vi "aparExecution_ModularLoop.vi"(9 "Motion Cfg File path":path=path "C:/Users/Public/Documents/UCAR/APAR Board Test/SupportFiles/Motion64.ini", 10 "Cfg File path":path=path "C:/Users/Public/Documents/UCAR/APAR Board Test/SupportFiles/aparConfig.ini", 11 "MessageQues":T1) -> ()   [LabVIEW 2017]
doc: "This VI is a simple state machine that has a message que so it can be controlled by external processes.\nIt also has a control with all the messages ques in the calling application that it needs to send messages to.\n\nThe concept is to have many parallel VIs like this one. This VI should be a cohesive process. This could cut down on it's size and complexity.\n\nBolder Software LLC"
uses:
  Support/MessageQue/VXM Main Test App/MultipleMessageQues vxm.ctl
  Support/MessageQue/MessageQue.ctl
  Support/MessageQue/MessageCluster.ctl
  Classes/aparCfg/aparCfg.lvclass
  Classes/ArrayController/ArrayController.lvclass
  Classes/N5222A PNA/N5222A PNA.lvclass
  Classes/Sequence/Sequence.lvclass
  Classes/Datalog/DataLog.lvclass
  Classes/SendMessage/SendMessage.lvclass
  Classes/MotionComm/MotionComm.lvclass
  Classes/FileMerge/FileMerge.lvclass
  C:/Users/Public/Documents/OU PAARD/mmWave_RF_Scanner/LVSource/Classes/Datalog/DataLog.lvclass
  Classes/DataLogRaster/DataLogRaster.lvclass
  Support/MessageAPI/UIMessage.ctl
  Support/MessageQue/MessageQue.lvlib
  Classes/VXMCfg/VXMCfg.lvclass
panel:
  out "Seq Step":string
  out "i":i32
  out "Command":string
  out "error out":errorcluster
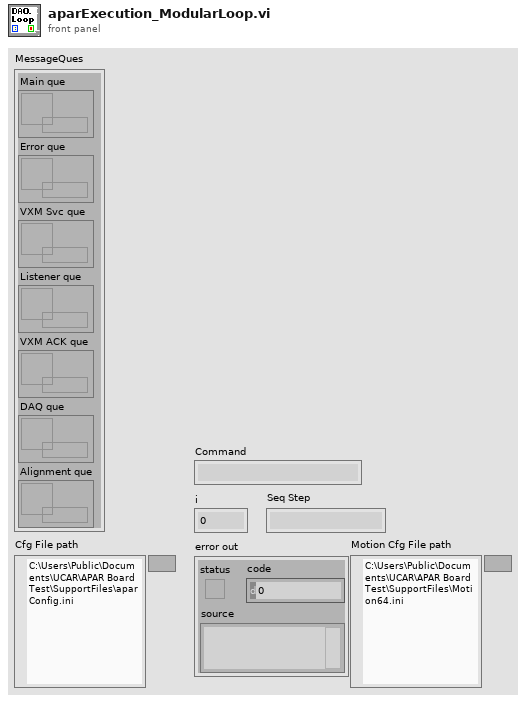
[diagram p1: front panel]
types:
  T1 = typedef "MultipleMessageQues vxm.ctl" = cluster{"Main que":T2, "Error que":T2, "VXM Svc que":T2, "Listener que":T2, "VXM ACK que":T2, "DAQ que":T2, "Alignment que":T2}
  T2 = typedef "MessageQue.lvlib/MessageQue.ctl" = refnum<queue>
  T3 = cluster{"aparCfg":refnum<class "aparCfg.lvclass">, "AC":refnum<class "ArrayController.lvclass">, "PNA":refnum<class "N5222A PNA.lvclass">, "Sequence":refnum<class "Sequence.lvclass">, "DataLog":refnum<class "DataLog.lvclass">, "UI Msg":refnum<class "SendMessage.lvclass">, "Motion ACK":refnum<class "MotionComm.lvclass">}
  T4 = typedef "UIMessage.ctl" = cluster{"EventCode":i32, "Numeric":dbl, "String":string, "Variant":variant}
  T5 = typedef "ACConfig.ctl" = cluster{"ACIPAddress":string, "timeout ms":i32, "AC (Dest.) port":u16, "Enable":bool}
  T6 = typedef "N5222AConfig.ctl" = cluster{"ResourceName":string, "Enable":bool, "Channel":i32, "CalFileName":string, "MeasName":string, "TempDatFile":string, "Power, dBm":dbl, "NumPoints":i32, "Start Freq, Hz":dbl, "Stop Freq, Hz":dbl, "NumAverages":i32, "Sweep Type":i32}
  T7 = typedef "seqConfig.ctl" = cluster{"TempXMLFilePath":path, "Motion":bool}
  T8 = typedef "RunTest.ctl" = cluster{"FileNameRoot":string, "MergeFilePath":path, "Merge":bool}
  T9 = typedef "DataLogConfig.ctl" = cluster{"FilePath":path}
  T10 = cluster{"X step":dbl, "Y step":dbl, "Z step":dbl, "T step":dbl}[]
  T11 = typedef "rasterConfig.ctl" = cluster{"Nyquist, mm":dbl, "Window, cm":dbl, "Polarization, V0 H1":T12, "RF Direction Tx0":T13}
  T12 = typedef "PolarizationSelect.ctl" = enum16{"Vertical", "Horizontal"}
  T13 = typedef "RF Direction.ctl" = enum16{"Tx - RF In", "Rx - RF Out"}
  T14 = typedef "DataLog.lvclass/SearchableTag.ctl" = cluster{"Module, 0-63":i32, "RF Direction Tx0":T13, "Polarization, V0 H1":T12, "PhaseShift, deg":dbl, "Atten, dB":dbl}
  T15 = typedef "PatchNewTestStep.ctl" = cluster{"RF In/Out":T13, "TR Module/Raster":i32, "Polarization":T12, "Position":cluster{"X mm":dbl, "Y mm":dbl, "Z mm":dbl, "T deg":dbl}}
  T16 = cluster{"X mm":dbl, "Y mm":dbl, "Z mm":dbl, "T deg":dbl}
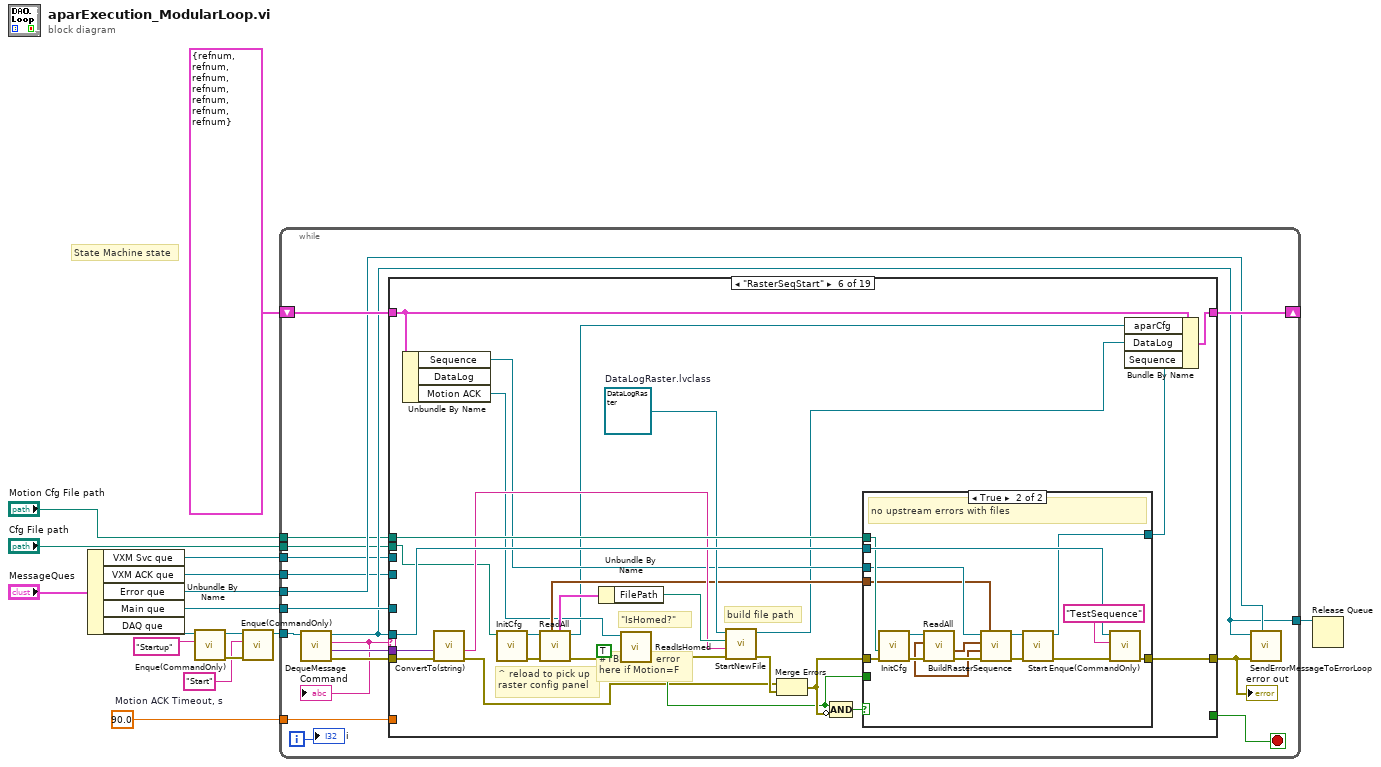
[diagram p0: block diagram]
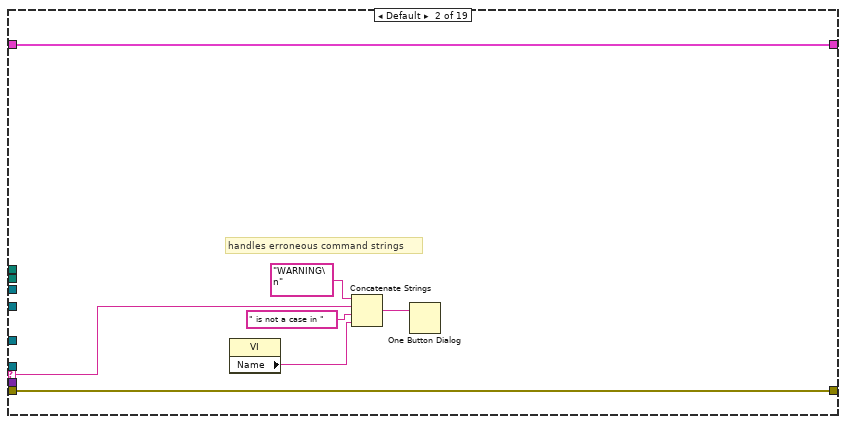
[diagram p3: hidden frame]
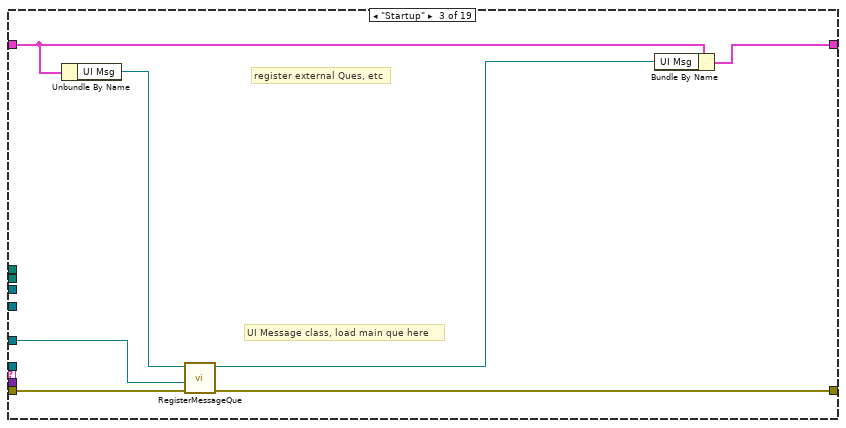
[diagram p4: hidden frame]
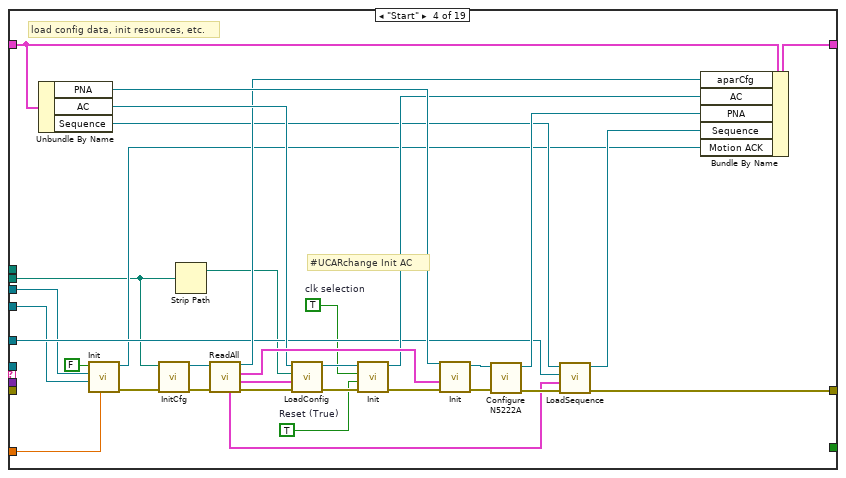
[diagram p5: hidden frame]
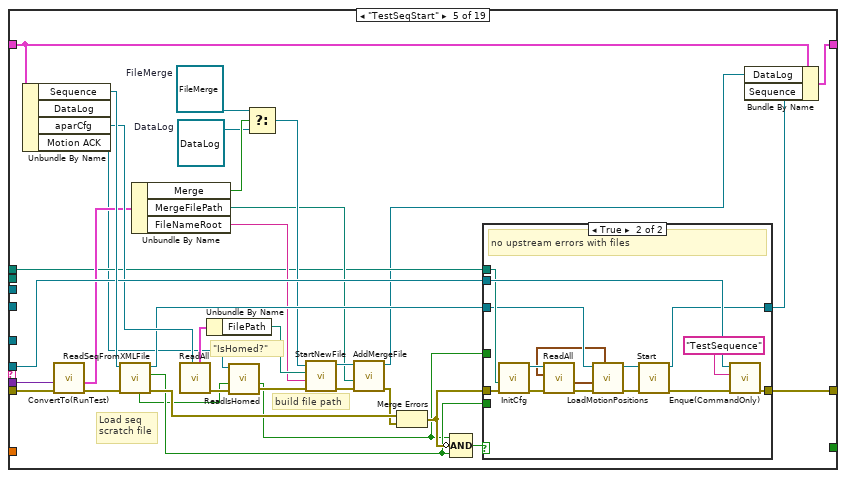
[diagram p6: hidden frame]
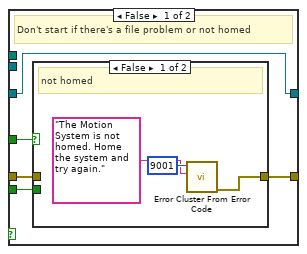
[diagram p7: hidden frame]
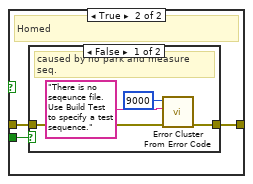
[diagram p8: hidden frame]
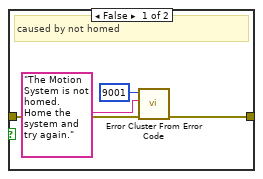
[diagram p11: hidden frame]
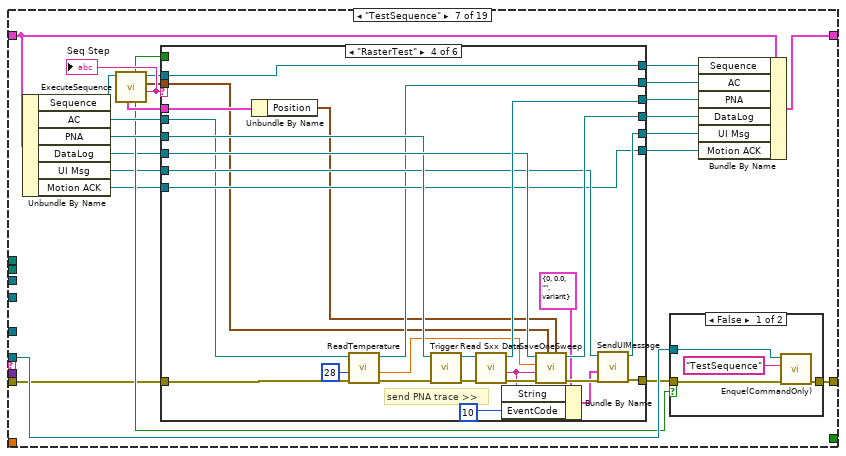
[diagram p12: hidden frame]
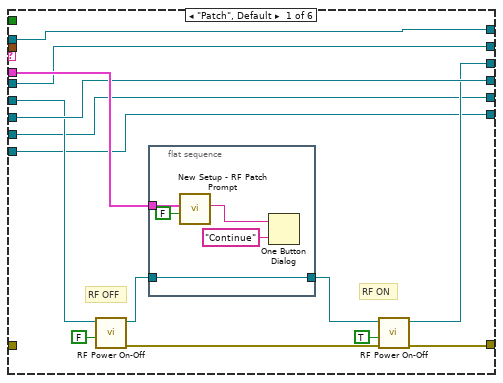
[diagram p13: hidden frame]
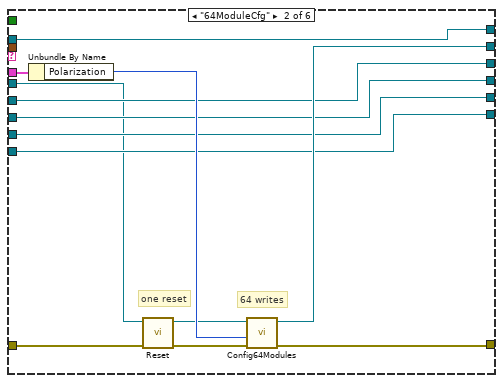
[diagram p14: hidden frame]
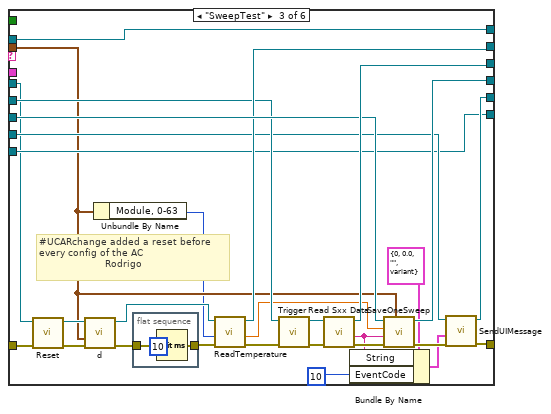
[diagram p15: hidden frame]
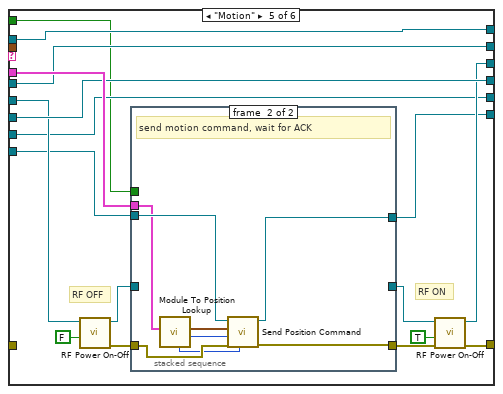
[diagram p16: hidden frame]
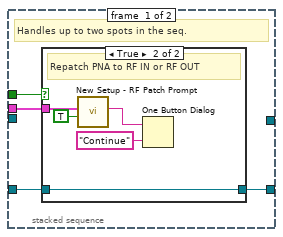
[diagram p17: hidden frame]
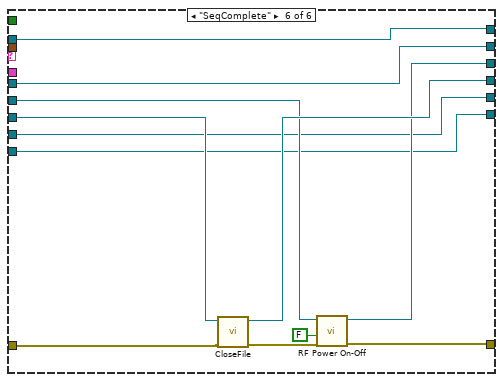
[diagram p19: hidden frame]
diagram:
  w2 = 90.0  # Motion ACK Timeout, s
  # "State Machine state"
  n1 = Unbundle By Name("MessageQues") -> ("VXM Svc que"=w4:T2, "VXM ACK que"=w3:T2, "Error que"=w14:T2, "Main que"=w15:T2, "DAQ que"=w12:T2)
  n2 = call "Enque(CommandOnly).vi"("Message Command"="Startup" ("Command"), "Message que"=w12) -> ("error out"=w9:errorcluster, "Message que out"=w8:T2)  [unwired: 8 in]
  n3 = call "Enque(CommandOnly).vi"("error in"=w9, "Message Command"="Start", "Message que"=w8) -> ("Message que out"=w7:T2)  [unwired: 7 in, 1 out]
  n4 = while {
    tunnel: w7 -> [w33]
    tunnel: w15 -> [w32]
    tunnel: w14 -> [w23]
    tunnel: [w22] -> w13
    shift-right: [w28] -> _
    shift-left: T3 {"aparCfg"=refnum, "AC"=refnum, "PNA"=refnum, "Sequence"=refnum, "DataLog"=refnum, "UI Msg"=refnum, "Motion ACK"=refnum} -> [w27]
    tunnel: "Cfg File path" -> [w21]
    tunnel: w4 -> [w20]
    tunnel: w3 -> [w19]
    tunnel: w2 -> [w18]
    tunnel: "Motion Cfg File path" -> [w17]
    i -> [w26]
    stop <- w30 stop-if-true
    n5 = call "DequeMessage.vi"("Message que"=w33) -> ("error out"=w31:errorcluster, "Message Payload"=w29:variant, "Message Command"=w25:string, "Message que out"=w22:T2)  [unwired: 5 in, 2 out]
    "Command" <- w25
    n6 = case shown="\"RasterSeqStart\"" w25 {
      selector: w25 -> [_ w36 _ _ _ _ _ _ _ _ _ _ _ _ _ _ _ _ _]
      tunnel: w32 -> [_ _ w43 w58 _ _ _ _ _ _ _ _ _ _ _ _ _ _ _]
      tunnel: w22 -> [_ _ _ _ w113 w173 w222 w365 w379 w393 w403 _ _ _ _ _ _ _ _]
      tunnel: [_ w41 w47 w62 w115 w174 w223 w372 w381 w400 w405 _ w415 w426 w436 w448 _ w458 _] -> w24
      tunnel: w31 -> [_ w41 w42 _ w109 w169 w208 w366 w382 w399 w404 _ w414 w431 w440 w448 _ _ _]
      tunnel: [_ _ _ _ _ _ _ _ _ _ _ _ _ _ _ _ _ _ TRUE] -> w30
      tunnel: w29 -> [_ _ _ _ w110 w170 _ _ _ _ _ _ _ w430 w444 _ _ w457 _]
      tunnel: [w34 w40 w45 w72 w111 w171 w218 w370 w386 w402 w412 w413 w417 w433 w438 w446 w455 w459 w460] -> w28
      tunnel: w27 -> [w34 w40 w46 w73 w112 w172 w219 w368 w384 w401 w412 w413 w418 w434 w439 w447 w456 w459 w460]
      tunnel: w21 -> [_ _ _ w50 _ w151 _ _ _ _ _ _ _ _ _ _ _ _ _]
      tunnel: w20 -> [_ _ _ w54 _ _ _ _ _ _ _ _ _ _ _ _ _ _ _]
      tunnel: w19 -> [_ _ _ w53 _ _ _ _ _ _ _ _ _ _ _ _ _ _ _]
      tunnel: w18 -> [_ _ _ w52 _ _ _ _ _ _ _ _ _ _ _ _ _ _ _]
      tunnel: w17 -> [_ _ _ _ w88 w163 _ _ _ _ _ _ _ _ _ _ _ _ _]
      frame "idle" {
      }
      frame Default {
        # "handles erroneous command strings"
        n7 = property class="VI"() -> ("Name"=w35:string)  [unwired: 2 in, 2 out]
        n8 = Concatenate Strings("WARNING\n" ("message"), w36, " is not a case in " ("message"), w35) -> (w39:string)
        n9 = One Button Dialog(message=w39) -> ()  [unwired: 1 in, 1 out]
      }
      frame "Startup" {
        # "UI Message class, load main que here"
        # "register external Ques, etc"
        n10 = Unbundle By Name(w46) -> ("UI Msg"=w48:refnum<class "SendMessage.lvclass">)
        n11 = call "RegisterMessageQue.vi"("error in (no error)"=w42, "Message que"=w43, "SendMessage in"=w48) -> ("error out"=w47:errorcluster, "SendMessage out"=w44:refnum<class "SendMessage.lvclass">)  [unwired: 7 in]
        n12 = Bundle By Name(cluster=w46, "UI Msg"=w44) -> (w45:T3)
      }
      frame "Start" {
        w51 = TRUE  # clk selection
        w64 = TRUE  # Reset (True)
        # "#UCARchange Init AC"
        # "load config data, init resources, etc."
        n13 = Unbundle By Name(w73) -> ("PNA"=w74:refnum<class "N5222A PNA.lvclass">, "AC"=w75:refnum<class "ArrayController.lvclass">, "Sequence"=w61:refnum<class "Sequence.lvclass">)
        n14 = call "Init.vi"("Timeout, s"=w52, "VXM ACK que"=w53, "VXM Svc que"=w54, "Standalone"=FALSE) -> ("error out"=w57:errorcluster, "MotionComm out"=w56:refnum<class "MotionComm.lvclass">)  [unwired: 6 in]
        n15 = call "InitCfg.vi"("error in (no error)"=w57, "Cfg File path"=w50) -> ("error out"=w68:errorcluster, "aparCfg out"=w69:refnum<class "aparCfg.lvclass">)  [unwired: 8 in]
        n16 = Strip Path(path=w50) -> (stripped path=w49:path)  [unwired: 1 out]
        n17 = call "ReadAll.vi"("error in (no error)"=w68, "aparCfg in"=w69) -> ("error out"=w77:errorcluster, "ACConfig"=w81:T5, "N5222A Cfg"=w79:T6, "aparCfg out"=w71:refnum<class "aparCfg.lvclass">, "SequenceConfig"=w59:T7)  [unwired: 3 in, 2 out]
        n18 = call "LoadConfig.vi"("error in (no error)"=w77, "AC Config"=w81, "Support Files Path"=w49, "ArrayController in"=w75) -> ("error out"=w80:errorcluster, "ArrayController out"=w76:refnum<class "ArrayController.lvclass">)  [unwired: 6 in]
        n19 = call "Init.vi"("error in (no error)"=w80, "Reset (True)"=w64, "clk selection"=w51, "ArrayController in"=w76) -> ("error out"=w78:errorcluster, "ArrayController out"=w70:refnum<class "ArrayController.lvclass">)  [unwired: 5 in, 1 out]
        n20 = call "Init.vi"("error in (no error)"=w78, "N5222A Cfg"=w79, "N5222A PNA in"=w74) -> ("error out"=w65:errorcluster, "N5222A PNA out"=w67:refnum<class "N5222A PNA.lvclass">)  [unwired: 7 in]
        n21 = call "Configure N5222A.vi"("error in (no error)"=w65, "N5222A PNA in"=w67) -> ("error out"=w63:errorcluster, "N5222A PNA out"=w66:refnum<class "N5222A PNA.lvclass">)  [unwired: 8 in]
        n22 = call "LoadSequence.vi"("error in (no error)"=w63, "Sequence Cfg"=w59, "Message que"=w58, "Sequence in"=w61) -> ("error out"=w62:errorcluster, "Sequence out"=w60:refnum<class "Sequence.lvclass">)  [unwired: 6 in]
        n23 = Bundle By Name(cluster=w73, "aparCfg"=w71, "AC"=w70, "PNA"=w66, "Sequence"=w60, "Motion ACK"=w56) -> (w72:T3)
      }
      frame "TestSeqStart" {
        w96 = refnum<class "FileMerge.lvclass"> refnum  # FileMerge
        w95 = refnum<class "DataLog.lvclass"> refnum  # DataLog
        # "\"IsHomed?\""
        # "build file path"
        # "Load seq \nscratch file"
        n24 = Unbundle By Name(w112) -> ("Sequence"=w114:refnum<class "Sequence.lvclass">, "aparCfg"=w107:refnum<class "aparCfg.lvclass">, "Motion ACK"=w84:refnum<class "MotionComm.lvclass">)  [unwired: 1 out]
        n25 = call "ConvertTo(RunTest).vi"("error in"=w109, "Message Payload"=w110) -> ("error out"=w108:errorcluster, "RunTest"=w106:T8)  [unwired: 8 in]
        n26 = call "ReadSeqFromXMLFile.vi"("error in (no error)"=w108, "Sequence in"=w114) -> ("error out"=w103:errorcluster, "Valid Seq"=w99:bool, "Sequence out"=w102:refnum<class "Sequence.lvclass">, "Motion"=w82:bool)  [unwired: 5 in, 1 out]
        n27 = Unbundle By Name(w106) -> ("Merge"=w97:bool, "MergeFilePath"=w89:path, "FileNameRoot"=w90:string)
        n28 = call "ReadAll.vi"("aparCfg in"=w107) -> ("error out"=w86:errorcluster, "DataLogConfig"=w105:T9)  [unwired: 4 in, 5 out]
        n29 = Unbundle By Name(w105) -> ("FilePath"=w104:path)
        n30 = call "ReadIsHomed.vi"("error in (no error)"=w86, "Motion Config"=w82, "MotionComm in"=w84) -> ("error out"=w85:errorcluster, "True = Homed"=w83:bool)  [unwired: 6 in, 1 out]
        n31 = Select(t=w96, s=w97, f=w95) -> (s? t:f=w94:refnum<class "DataLog.lvclass">)
        n32 = call-dynamic "StartNewFile.vi"("error in (no error)"=w85, "Root File Name"=w90, "Data Files Folder Path"=w104, "DataLog in"=w94) -> ("error out"=w93:errorcluster, "DataLog out"=w91:refnum<class "DataLog.lvclass">)  [unwired: 6 in]
        n33 = call-dynamic "AddMergeFile.vi"("error in (no error)"=w93, "ExistingFilePath"=w89, "DataLog in"=w91) -> ("error out"=w92:errorcluster, "DataLog out"=w87:refnum<class "DataLog.lvclass">)  [unwired: 7 in]
        n34 = Merge Errors(w103, w92) -> (w101:errorcluster)
        n35 = Compound Arithmetic op=AND(w83, invert w101, w99) -> (w100:bool)
        n36 = case shown="True" w100 {
          tunnel: [w119 w146] -> w115
          tunnel: w113 -> [_ w145]
          tunnel: w101 -> [w120 w140]
          tunnel: w102 -> [w117 w134]
          tunnel: [w117 w142] -> w98
          tunnel: w99 -> [w118 _]
          tunnel: w88 -> [_ w138]
          tunnel: w83 -> [w116 _]
          frame False {
            # "Don't start if there's a file problem or not homed"
            n37 = case shown="False" w116 {
              tunnel: w120 -> [_ w126]
              tunnel: [w121 w125] -> w119
              tunnel: w118 -> [_ w124]
              frame False {
                # "not homed"
                n38 = call <vilib>:"Error Cluster From Error Code.vi"("error message (\"\")"="The Motion System is not homed. Home the system and try again." ("error message (\"\")"), "error code (0)"=9001) -> ("error out"=w121:errorcluster)  [unwired: 7 in]
              }
              frame True {
                # "Homed"
                n39 = case shown="False" w124 {
                  tunnel: w126 -> [w130 w131]
                  tunnel: [w129 w131] -> w125
                  frame False {
                    # "caused by no park and measure seq."
                    n40 = call <vilib>:"Error Cluster From Error Code.vi"("error in (no error)"=w130, "error message (\"\")"="There is no seqeunce file. Use Build Test to specify a test sequence." ("error message (\"\")"), "error code (0)"=9000) -> ("error out"=w129:errorcluster)  [unwired: 6 in]
                  }
                  frame True {
                    # "pass through error"
                  }
                }
              }
            }
          }
          frame True {
            # "no upstream errors with files"
            n41 = call "InitCfg.vi"("error in (no error)"=w140, "Cfg File path"=w138) -> ("error out"=w139:errorcluster, "VXMCfg out"=w141:refnum<class "VXMCfg.lvclass">)  [unwired: 7 in, 1 out]
            n42 = call "ReadAll.vi"("error in (no error)"=w139, "VXMCfg in"=w141) -> ("error out"=w137:errorcluster, "Position Array"=w133:T10, "TestZT"=w132:cluster{"Z mm":dbl, "Horizontal T deg":dbl})  [unwired: 7 out]
            n43 = call "LoadMotionPositions.vi"("TestZT"=w132, "error in (no error)"=w137, "Position Array"=w133, "Sequence in"=w134) -> ("error out"=w136:errorcluster, "Sequence out"=w135:refnum<class "Sequence.lvclass">)  [unwired: 6 in]
            n44 = call "Start.vi"("error in (no error)"=w136, "Sequence in"=w135) -> ("error out"=w143:errorcluster, "Sequence out"=w142:refnum<class "Sequence.lvclass">)  [unwired: 8 in]
            n45 = call "Enque(CommandOnly).vi"("error in"=w143, "Message Command"="TestSequence" ("Command"), "Message que"=w145) -> ("error out"=w146:errorcluster)  [unwired: 7 in, 1 out]
          }
        }
        n46 = Bundle By Name(cluster=w112, "DataLog"=w87, "Sequence"=w98) -> (w111:T3)
      }
      frame "RasterSeqStart" {
        w159 = refnum<class "DataLogRaster.lvclass"> refnum  # DataLogRaster.lvclass
        # "#TBD need error here if Motion=F"
        # "^ reload to pick up\nraster config panel"
        # "\"IsHomed?\""
        # "build file path"
        n47 = Unbundle By Name(w172) -> ("Sequence"=w156:refnum<class "Sequence.lvclass">, "Motion ACK"=w152:refnum<class "MotionComm.lvclass">)  [unwired: 1 out]
        n48 = call "ConvertTo(string).vi"("error in"=w169, "Message Payload"=w170) -> ("error out"=w148:errorcluster, "Message Payload string"=w160:string)  [unwired: 8 in]
        n49 = call "InitCfg.vi"("Cfg File path"=w151) -> ("error out"=w149:errorcluster, "aparCfg out"=w153:refnum<class "aparCfg.lvclass">)  [unwired: 9 in]
        n50 = call "ReadAll.vi"("error in (no error)"=w149, "aparCfg in"=w153) -> ("error out"=w162:errorcluster, "aparCfg out"=w150:refnum<class "aparCfg.lvclass">, "DataLogConfig"=w168:T9, "apar properties.RasterDef"=w155:T11)  [unwired: 3 in, 3 out]
        n51 = Unbundle By Name(w168) -> ("FilePath"=w167:path)
        n52 = call "ReadIsHomed.vi"("error in (no error)"=w162, "Motion Config"=TRUE, "MotionComm in"=w152) -> ("error out"=w161:errorcluster, "True = Homed"=w157:bool)  [unwired: 6 in, 1 out]
        n53 = call-dynamic "StartNewFile.vi"("error in (no error)"=w161, "Root File Name"=w160, "Data Files Folder Path"=w167, "DataLogRaster in"=w159) -> ("error out"=w158:errorcluster, "DataLogRaster out"=w154:refnum<class "DataLogRaster.lvclass">)  [unwired: 6 in]
        n54 = Merge Errors(w148, w158) -> (w166:errorcluster)
        n55 = Compound Arithmetic op=AND(w157, invert w166) -> (w165:bool)
        n56 = case shown="True" w165 {
          tunnel: [w177 w199] -> w174
          tunnel: w173 -> [_ w198]
          tunnel: w166 -> [w178 w195]
          tunnel: w156 -> [w175 w191]
          tunnel: [w175 w184] -> w164
          tunnel: w157 -> [w176 _]
          tunnel: w163 -> [_ w193]
          tunnel: w155 -> [_ w188]
          frame False {
            # "Don't start if there's a file problem or not homed"
            n57 = case shown="True" w176 {
              tunnel: w178 -> [w182 w183]
              tunnel: [w181 w183] -> w177
              frame False {
                # "caused by not homed"
                n58 = call <vilib>:"Error Cluster From Error Code.vi"("error in (no error)"=w182, "error message (\"\")"="The Motion System is not homed. Home the system and try again." ("error message (\"\")"), "error code (0)"=9001) -> ("error out"=w181:errorcluster)  [unwired: 6 in]
              }
              frame True {
                # "pass through error"
              }
            }
          }
          frame True {
            # "no upstream errors with files"
            n59 = call "InitCfg.vi"("error in (no error)"=w195, "Cfg File path"=w193) -> ("error out"=w194:errorcluster, "VXMCfg out"=w196:refnum<class "VXMCfg.lvclass">)  [unwired: 7 in, 1 out]
            n60 = call "ReadAll.vi"("error in (no error)"=w194, "VXMCfg in"=w196) -> ("error out"=w192:errorcluster, "Position Array"=w190:T10, "TestZT"=w189:cluster{"Z mm":dbl, "Horizontal T deg":dbl})  [unwired: 7 out]
            n61 = call "BuildRasterSequence.vi"("RasterDef"=w188, "error in (no error)"=w192, "TestZT"=w189, "Position Array in"=w190, "Sequence in"=w191) -> ("error out"=w186:errorcluster, "Sequence out"=w187:refnum<class "Sequence.lvclass">)  [unwired: 4 in, 1 out]
            n62 = call "Start.vi"("error in (no error)"=w186, "Sequence in"=w187) -> ("error out"=w185:errorcluster, "Sequence out"=w184:refnum<class "Sequence.lvclass">)  [unwired: 8 in]
            n63 = call "Enque(CommandOnly).vi"("error in"=w185, "Message Command"="TestSequence" ("Command"), "Message que"=w198) -> ("error out"=w199:errorcluster)  [unwired: 7 in, 1 out]
          }
        }
        n64 = Bundle By Name(cluster=w172, "aparCfg"=w150, "DataLog"=w154, "Sequence"=w164) -> (w171:T3)
      }
      frame "TestSequence" {
        n65 = Unbundle By Name(w219) -> ("Sequence"=w221:refnum<class "Sequence.lvclass">, "AC"=w214:refnum<class "ArrayController.lvclass">, "PNA"=w212:refnum<class "N5222A PNA.lvclass">, "DataLog"=w205:refnum<class "DataLog.lvclass">, "UI Msg"=w204:refnum<class "SendMessage.lvclass">, "Motion ACK"=w201:refnum<class "MotionComm.lvclass">)
        n66 = call "ExecuteSequence.vi"("Sequence in"=w221) -> ("Command"=w220:string, "SweepProperties"=w211:T14, "Sequence out"=w217:refnum<class "Sequence.lvclass">, "Sequence is done"=w209:bool, "Prompt Operator RF In/Out"=w202:bool, "NewSetup"=w210:T15)  [unwired: 4 in, 1 out]
        "Seq Step" <- w220
        n67 = case shown="\"RasterTest\"" w220 {
          tunnel: [w235 w255 w284 w312 w327 w359] -> w216
          tunnel: w217 -> [w235 w255 w284 w312 w327 w359]
          tunnel: [w236 w253 w275 w292 w328 w358] -> w215
          tunnel: w214 -> [w236 w243 w259 w293 w328 w358]
          tunnel: [w226 w250 w281 w309 w321 w351] -> w213
          tunnel: w212 -> [w227 w250 w272 w305 w322 w352]
          tunnel: w211 -> [_ _ w257 w288 _ _]
          tunnel: w210 -> [w237 w252 _ w290 w329 _]
          tunnel: w208 -> [_ w245 w261 w294 _ w357]
          tunnel: [w229 w254 w269 w303 w324 w350] -> w207
          tunnel: [w228 w249 w277 w306 w323 w355] -> w206
          tunnel: w205 -> [w228 w249 w278 w307 w323 w356]
          tunnel: w204 -> [w225 w248 w268 w302 w320 w349]
          tunnel: [w225 w248 w267 w301 w320 w349] -> w203
          tunnel: w202 -> [_ _ _ _ w317 _]
          tunnel: w201 -> [w224 w247 w262 w296 w314 w348]
          tunnel: [w224 w247 w262 w296 w313 w348] -> w200
          frame "Patch", Default {
            # "RF ON"
            # "RF OFF"
            n68 = call "RF Power On-Off.vi"("RF Power State (T: On)"=FALSE, "N5222A PNA in"=w227) -> ("error out"=w232:errorcluster, "N5222A PNA out"=w231:refnum<class "N5222A PNA.lvclass">)  [unwired: 8 in]
            n69 = flat-sequence {
              tunnel: w237 -> [w240]
              tunnel: [w239] -> w230
              tunnel: w231 -> [w239]
              frame #0 {
                n70 = call "New Setup - RF Patch Prompt.vi"("Motion"=FALSE, "NewSetup"=w240) -> ("Dialog Prompt"=w241:string)  [unwired: 9 in]
                n71 = One Button Dialog(message=w241, button name ("OK")="Continue") -> ()  [unwired: 1 out]
              }
            }
            n72 = call "RF Power On-Off.vi"("error in (no error)"=w232, "RF Power State (T: On)"=TRUE, "N5222A PNA in"=w230) -> ("error out"=w229:errorcluster, "N5222A PNA out"=w226:refnum<class "N5222A PNA.lvclass">)  [unwired: 7 in]
          }
          frame "64ModuleCfg" {
            # "one reset"
            # "64 writes"
            n73 = Unbundle By Name(w252) -> ("Polarization"=w251:T12)
            n74 = call "Reset.vi"("error in (no error)"=w245, "ArrayController in"=w243) -> ("error out"=w244:errorcluster, "ArrayController out"=w246:refnum<class "ArrayController.lvclass">)  [unwired: 8 in]
            n75 = call "Config64Modules.vi"("error in (no error)"=w244, "Polarization"=w251, "ArrayController in"=w246) -> ("error out"=w254:errorcluster, "ArrayController out"=w253:refnum<class "ArrayController.lvclass">)  [unwired: 7 in]
          }
          frame "SweepTest" {
            # "#UCARchange added a reset before\nevery config of the AC\n                      Rodrigo"
            n76 = call "Reset.vi"("error in (no error)"=w261, "ArrayController in"=w259) -> ("error out"=w260:errorcluster, "ArrayController out"=w258:refnum<class "ArrayController.lvclass">)  [unwired: 8 in]
            n77 = call "d.vi"("error in (no error)"=w260, "d Cmd Properties"=w257, "ArrayController in"=w258) -> ("error out"=w280:errorcluster, "ArrayController out"=w276:refnum<class "ArrayController.lvclass">)  [unwired: 7 in]
            n78 = Unbundle By Name(w257) -> ("Module, 0-63"=w256:i32)
            n79 = flat-sequence {
              tunnel: [w285] -> w273
              tunnel: w280 -> [w285]
              frame #0 {
                n80 = Wait (ms)(milliseconds to wait=u32 10) -> ()  [unwired: 1 out]
              }
            }
            n81 = call "ReadTemperature.vi"("error in (no error)"=w273, "Module Number (0-63)"=w256, "ArrayController in"=w276) -> ("error out"=w274:errorcluster, "Temp, deg C"=w271:dbl, "ArrayController out"=w275:refnum<class "ArrayController.lvclass">)  [unwired: 6 in]
            n82 = call "Trigger.vi"("error in (no error)"=w274, "N5222A PNA in"=w272) -> ("error out"=w283:errorcluster, "N5222A PNA out"=w282:refnum<class "N5222A PNA.lvclass">)  [unwired: 8 in]
            n83 = call "Read Sxx Data.vi"("error in (no error)"=w283, "N5222A PNA in"=w282) -> ("error out"=w279:errorcluster, ".csv file"=w263:string, "N5222A PNA out"=w281:refnum<class "N5222A PNA.lvclass">)  [unwired: 7 in]
            n84 = Bundle By Name(cluster=T4 {"EventCode"=0, "Numeric"=0.0, "String"="", "Variant"=variant} ("UIMsg"), "String"=w263, "EventCode"=10) -> (w265:T4)
            n85 = call-dynamic "SaveOneSweep.vi"("SectionProperties"=w257, "error in (no error)"=w279, ".csv file from N5222A"=w263, "Temperature, deg C"=w271, "DataLog in"=w278) -> ("error out"=w270:errorcluster, "DataLog out"=w277:refnum<class "DataLog.lvclass">)  [unwired: 5 in]
            n86 = call-dynamic "SendUIMessage.vi"("error in (no error)"=w270, "UIMsg"=w265, "SendMessage in"=w268) -> ("error out"=w269:errorcluster, "SendMessage out"=w267:refnum<class "SendMessage.lvclass">)  [unwired: 7 in]
          }
          frame "RasterTest" {
            # "send PNA trace >>"
            n87 = Unbundle By Name(w290) -> ("Position"=w289:T16)
            n88 = call "ReadTemperature.vi"("error in (no error)"=w294, "Module Number (0-63)"=28, "ArrayController in"=w293) -> ("error out"=w295:errorcluster, "Temp, deg C"=w291:dbl, "ArrayController out"=w292:refnum<class "ArrayController.lvclass">)  [unwired: 6 in]
            n89 = call "Trigger.vi"("error in (no error)"=w295, "N5222A PNA in"=w305) -> ("error out"=w311:errorcluster, "N5222A PNA out"=w310:refnum<class "N5222A PNA.lvclass">)  [unwired: 8 in]
            n90 = call "Read Sxx Data.vi"("error in (no error)"=w311, "N5222A PNA in"=w310) -> ("error out"=w308:errorcluster, ".csv file"=w297:string, "N5222A PNA out"=w309:refnum<class "N5222A PNA.lvclass">)  [unwired: 7 in]
            n91 = Bundle By Name(cluster=T4 {"EventCode"=0, "Numeric"=0.0, "String"="", "Variant"=variant} ("UIMsg"), "String"=w297, "EventCode"=10) -> (w299:T4)
            n92 = call-dynamic "SaveOneSweep.vi"("Position"=w289, "SectionProperties"=w288, "error in (no error)"=w308, ".csv file from N5222A"=w297, "Temperature, deg C"=w291, "DataLog in"=w307) -> ("error out"=w304:errorcluster, "DataLog out"=w306:refnum<class "DataLog.lvclass">)  [unwired: 4 in]
            n93 = call-dynamic "SendUIMessage.vi"("error in (no error)"=w304, "UIMsg"=w299, "SendMessage in"=w302) -> ("error out"=w303:errorcluster, "SendMessage out"=w301:refnum<class "SendMessage.lvclass">)  [unwired: 7 in]
          }
          frame "Motion" {
            # "RF ON"
            # "RF OFF"
            n94 = call "RF Power On-Off.vi"("RF Power State (T: On)"=FALSE, "N5222A PNA in"=w322) -> ("error out"=w316:errorcluster, "N5222A PNA out"=w319:refnum<class "N5222A PNA.lvclass">)  [unwired: 8 in]
            n95 = stacked-sequence {
              tunnel: w329 -> [w333 w342]
              tunnel: w319 -> [w332 _]
              tunnel: [w331 _] -> w318
              tunnel: w317 -> [w330 _]
              tunnel: [_ w347] -> w315
              tunnel: w316 -> [_ w343]
              tunnel: w314 -> [_ w346]
              tunnel: [_ w345] -> w313
              frame #0 {
                # "Handles up to two spots in the seq."
                n96 = case shown="True" w330 {
                  tunnel: w333 -> [_ w339]
                  tunnel: [w334 w335] -> w331
                  tunnel: w332 -> [w334 w335]
                  frame False {
                    # "motion handles \"repatch\""
                  }
                  frame True {
                    # "Repatch PNA to RF IN or RF OUT"
                    n97 = call "New Setup - RF Patch Prompt.vi"("Motion"=TRUE, "NewSetup"=w339) -> ("Dialog Prompt"=w337:string)  [unwired: 9 in]
                    n98 = One Button Dialog(message=w337, button name ("OK")="Continue") -> ()  [unwired: 1 out]
                  }
                }
              }
              frame #1 {
                # "send motion command, wait for ACK"
                n99 = call "Module To Position Lookup.vi"("NewSetup"=w342) -> ("TR Module/Raster num"=w341:i32, "Position"=w344:T16, "Polarization"=w340:u16)  [unwired: 8 in]
                n100 = call "Send Position Command.vi"("Polarization"=w340, "error in (no error)"=w343, "TR Module/Raster num"=w341, "Position"=w344, "MotionComm in"=w346) -> ("error out"=w347:errorcluster, "MotionComm out"=w345:refnum<class "MotionComm.lvclass">)  [unwired: 5 in]
              }
            }
            n101 = call "RF Power On-Off.vi"("error in (no error)"=w315, "RF Power State (T: On)"=TRUE, "N5222A PNA in"=w318) -> ("error out"=w324:errorcluster, "N5222A PNA out"=w321:refnum<class "N5222A PNA.lvclass">)  [unwired: 7 in]
          }
          frame "SeqComplete" {
            n102 = call-dynamic "CloseFile.vi"("error in (no error)"=w357, "DataLog in"=w356) -> ("error out"=w354:errorcluster, "DataLog out"=w355:refnum<class "DataLog.lvclass">)  [unwired: 8 in]
            n103 = call "RF Power On-Off.vi"("error in (no error)"=w354, "RF Power State (T: On)"=FALSE, "N5222A PNA in"=w352) -> ("error out"=w350:errorcluster, "N5222A PNA out"=w351:refnum<class "N5222A PNA.lvclass">)  [unwired: 7 in]
          }
        }
        n104 = case shown="False" w209 {
          tunnel: [w362 w364] -> w223
          tunnel: w222 -> [w361 _]
          tunnel: w207 -> [w360 w364]
          frame False {
            n105 = call "Enque(CommandOnly).vi"("error in"=w360, "Message Command"="TestSequence" ("Command"), "Message que"=w361) -> ("error out"=w362:errorcluster)  [unwired: 7 in, 1 out]
          }
          frame True {
          }
        }
        n106 = Bundle By Name(cluster=w219, "Sequence"=w216, "AC"=w215, "PNA"=w213, "DataLog"=w206, "UI Msg"=w203, "Motion ACK"=w200) -> (w218:T3)
      }
      frame "TestSeqPause" {
        n107 = Unbundle By Name(w368) -> ("Sequence"=w367:refnum<class "Sequence.lvclass">)
        n108 = call "Pause.vi"("error in (no error)"=w366, "Sequence in"=w367) -> ("error out"=w373:errorcluster, "SeqPaused"=w371:bool, "Sequence out"=w369:refnum<class "Sequence.lvclass">)  [unwired: 7 in]
        n109 = case shown="True" w371 {
          tunnel: [w374 w376] -> w372
          tunnel: w373 -> [w374 w377]
          tunnel: w365 -> [_ w375]
          frame False {
          }
          frame True {
            # "state becomes idle"
            n110 = Flush Queue(queue=w375, error in (no error)=w377) -> (error out=w376:errorcluster)  [unwired: 2 out]
          }
        }
        n111 = Bundle By Name(cluster=w368, "Sequence"=w369) -> (w370:T3)
      }
      frame "TestSeqResume" {
        n112 = Unbundle By Name(w384) -> ("Sequence"=w383:refnum<class "Sequence.lvclass">)
        n113 = call "Resume.vi"("error in (no error)"=w382, "Sequence in"=w383) -> ("error out"=w378:errorcluster, "TestSeqResumed"=w380:bool, "Sequence out"=w385:refnum<class "Sequence.lvclass">)  [unwired: 7 in]
        n114 = case shown="True" w380 {
          tunnel: [w387 w390] -> w381
          tunnel: w379 -> [_ w389]
          tunnel: w378 -> [w387 w388]
          frame False {
          }
          frame True {
            n115 = call "Enque(CommandOnly).vi"("error in"=w388, "Message Command"="TestSequence" ("Command"), "Message que"=w389) -> ("error out"=w390:errorcluster)  [unwired: 7 in, 1 out]
          }
        }
        n116 = Bundle By Name(cluster=w384, "Sequence"=w385) -> (w386:T3)
      }
      frame "TestSeqStop" {
        # "resume\nexecution"
        n117 = Unbundle By Name(w401) -> ("Sequence"=w398:refnum<class "Sequence.lvclass">)
        n118 = call "Stop.vi"("error in (no error)"=w399, "Sequence in"=w398) -> ("error out"=w395:errorcluster, "Sequence out"=w397:refnum<class "Sequence.lvclass">)  [unwired: 8 in]
        n119 = Flush Queue(queue=w393, error in (no error)=w395) -> (queue out=w392:T2, error out=w394:errorcluster)  [unwired: 1 out]
        n120 = Bundle By Name(cluster=w401, "Sequence"=w397) -> (w402:T3)
        n121 = call "Enque(CommandOnly).vi"("error in"=w394, "Message Command"="TestSequence" ("Command"), "Message que"=w392) -> ("error out"=w400:errorcluster)  [unwired: 7 in, 1 out]
      }
      frame "Restart" {
        # "load config data, init resources, etc."
        n122 = Flush Queue(queue=w403, error in (no error)=w404) -> (queue out=w406:T2, error out=w411:errorcluster)  [unwired: 1 out]
        n123 = call "Enque(CommandOnly).vi"("error in"=w411, "Message Command"="Stop_Close" ("Command"), "Message que"=w406) -> ("error out"=w410:errorcluster, "Message que out"=w408:T2)  [unwired: 7 in]
        n124 = call "Enque(CommandOnly).vi"("error in"=w410, "Message Command"="Start" ("Command"), "Message que"=w408) -> ("error out"=w405:errorcluster)  [unwired: 7 in, 1 out]
      }
      frame "Test" {
        # "should generate error if\nsettings or hardware are wrong"
      }
      frame "AC_Reset" {
        n125 = Unbundle By Name(w418) -> ("AC"=w419:refnum<class "ArrayController.lvclass">)
        n126 = call "Reset.vi"("error in (no error)"=w414, "ArrayController in"=w419) -> ("error out"=w415:errorcluster, "ArrayController out"=w416:refnum<class "ArrayController.lvclass">)  [unwired: 8 in]
        n127 = Bundle By Name(cluster=w418, "AC"=w416) -> (w417:T3)
      }
      frame "AC_Temperature" {
        n128 = call "ConvertTo(DBL).vi"("error in"=w431, "Message Payload"=w430) -> ("error out"=w429:errorcluster, "Message Payload DBL Numeric"=w428:dbl)  [unwired: 8 in]
        n129 = Unbundle By Name(w434) -> ("UI Msg"=w421:refnum<class "SendMessage.lvclass">, "AC"=w435:refnum<class "ArrayController.lvclass">)
        n130 = call "ReadTemperature.vi"("error in (no error)"=w429, "Module Number (0-63)"=w428, "ArrayController in"=w435) -> ("error out"=w427:errorcluster, "Temp, deg C"=w422:dbl, "ArrayController out"=w432:refnum<class "ArrayController.lvclass">)  [unwired: 6 in]
        n131 = Bundle By Name(cluster=T4 {"EventCode"=0, "Numeric"=0.0, "String"="", "Variant"=variant} ("UIMsg"), "EventCode"=8, "Numeric"=w422) -> (w423:T4)
        n132 = call-dynamic "SendUIMessage.vi"("error in (no error)"=w427, "UIMsg"=w423, "SendMessage in"=w421) -> ("error out"=w426:errorcluster, "SendMessage out"=w420:refnum<class "SendMessage.lvclass">)  [unwired: 7 in]
        n133 = Bundle By Name(cluster=w434, "AC"=w432, "UI Msg"=w420) -> (w433:T3)
      }
      frame "AC_d" {
        n134 = call "ConvertTo(waveform).vi"("error in"=w440, "Message Payload"=w444) -> ("error out"=w441:errorcluster, "d Cmd Payload"=w443:T14)  [unwired: 8 in]
        n135 = Unbundle By Name(w439) -> ("AC"=w442:refnum<class "ArrayController.lvclass">)
        n136 = call "d.vi"("error in (no error)"=w441, "d Cmd Properties"=w443, "ArrayController in"=w442) -> ("error out"=w436:errorcluster, "ArrayController out"=w437:refnum<class "ArrayController.lvclass">)  [unwired: 7 in]
        n137 = Bundle By Name(cluster=w439, "AC"=w437) -> (w438:T3)
      }
      frame "N5222A_Sweep" {
        n138 = Unbundle By Name(w447) -> ("PNA"=w445:refnum<class "N5222A PNA.lvclass">)
        n139 = Bundle By Name(cluster=w447, "PNA"=w445) -> (w446:T3)
      }
      frame "Stop_Close" {
        # "ignore errors"
        n140 = Unbundle By Name(w456) -> ("AC"=w453:refnum<class "ArrayController.lvclass">, "PNA"=w454:refnum<class "N5222A PNA.lvclass">)
        n141 = call "Close.vi"("N5222A PNA in"=w454) -> ("error out"=w451:errorcluster, "N5222A PNA out"=w450:refnum<class "N5222A PNA.lvclass">)  [unwired: 9 in]
        n142 = call "Close.vi"("ArrayController in"=w453) -> ("error out"=w452:errorcluster, "ArrayController out"=w449:refnum<class "ArrayController.lvclass">)  [unwired: 9 in]
        n143 = flat-sequence {
          tunnel: w452 -> [_]
          tunnel: w451 -> [_]
          frame #0 {
          }
        }
        n144 = Bundle By Name(cluster=w456, "PNA"=w450, "AC"=w449) -> (w455:T3)
      }
      frame "GenerateTestError" {
        n145 = call "ConvertTo(error).vi"("Message Payload"=w457) -> ("Message Payload error"=w458:errorcluster)  [unwired: 9 in, 1 out]
      }
      frame "ExitNow" {
      }
    }
    "error out" <- w24
    n146 = call "SendErrorMessageToErrorLoop.vi"("Error Message que"=w23, "error in (no error)"=w24, "Loop Message que"=w22) -> ()  [unwired: 8 in, 1 out]
    "i" <- w26
  }
  n147 = Release Queue(queue=w13) -> ()  [unwired: 2 in, 3 out]
